vi "schedule.vi"(6 "Lighting Power Consume (W)":dbl format="%#_13g", 8 "Lenght of Light Period (hr)":i32, 9 "Start Time of Light Period":i32, 10 "input envTemp. & elecFee":cluster{"Temp.":dbl[], "elecFee":dbl[]}={"Temp."=[29.6, 26.5, 26.8, 26.8, 26.5, 26.9, 27.8, 28.5, 26.3, 30.1, 33.3, 33.4, 33.9, 32.2, 32.7, 32.7, 32.4, 31.5, 30.5, 29.7, 28.3, 28.2, 27.9, 27.5], "elecFee"=[2.2, 2.2, 2.2, 2.2, 2.2, 2.2, 2.2, 2.2, 3.5, 3.5, 3.5, 3.5, 3.5, 3.5, 3.5, 3.5, 3.5, 3.5, 3.5, 3.5, 3.5, 3.5, 2.2, 2.2]}, 11 "input Parameter":T2={"input COP of ACs"=3.0, "input setDay Temp"=22.0, "input setNight Temp."=20.0}) -> (3 "group Outcome":T1 {"group hourly total elecFee" format="%#.2g"; "group Total elecFee" format="%#.2g"; "group hourly ACs elecFee" format="%#.2g"; "group ACs elecFee" format="%#.2g"; "group hourly LEDs elecFee" format="%#.2g"; "group Total LEDs elecFee" format="%#.2g"})   [LabVIEW 2014]
panel:
  out "setNight Temp.":dbl
  out "setDay Temp.":dbl
  out "COP of ACs":dbl
  # "0~1"
  # "1~2"
  # "2~3"
  # "3~4"
  # "4~5"
  # "5~6"
  # "6~7"
  # "7~8"
  # "8~98~9"
  # "9~10"
  # "10~11"
  # "11~12"
  # "12~13"
  # "13~14"
  # "14~15"
  # "15~16"
  # "16~17"
  # "17~18"
  # "18~19"
  # "19~20"
  # "21~21"
  # "21~22"
  # "22~23"
  # "23~24"
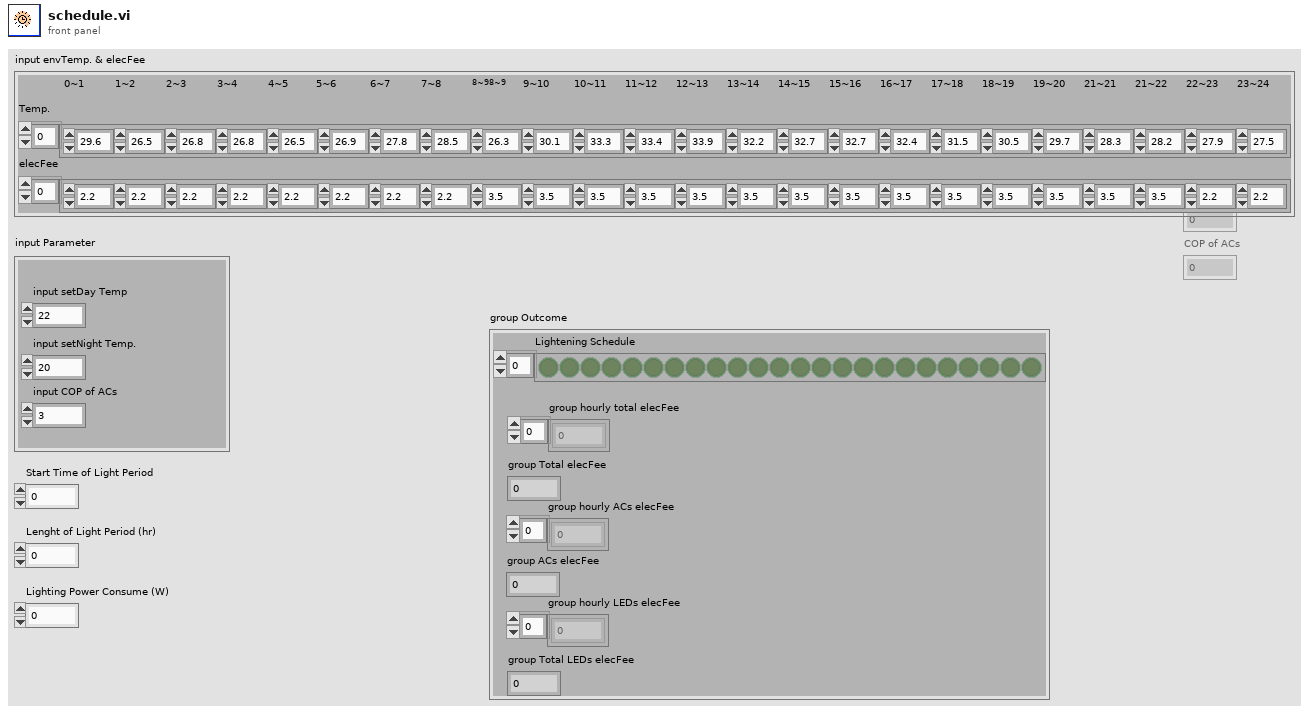
[diagram p1: front panel]
types:
  T1 = cluster{"Lightening Schedule":bool[], "group hourly total elecFee":dbl[], "group Total elecFee":dbl, "group hourly ACs elecFee":dbl[], "group ACs elecFee":dbl, "group hourly LEDs elecFee":dbl[], "group Total LEDs elecFee":dbl}
  T2 = cluster{"input COP of ACs":dbl, "input setDay Temp":dbl, "input setNight Temp.":dbl}
  T3 = cluster{bool[], dbl[], dbl, dbl[], dbl, dbl[], dbl}
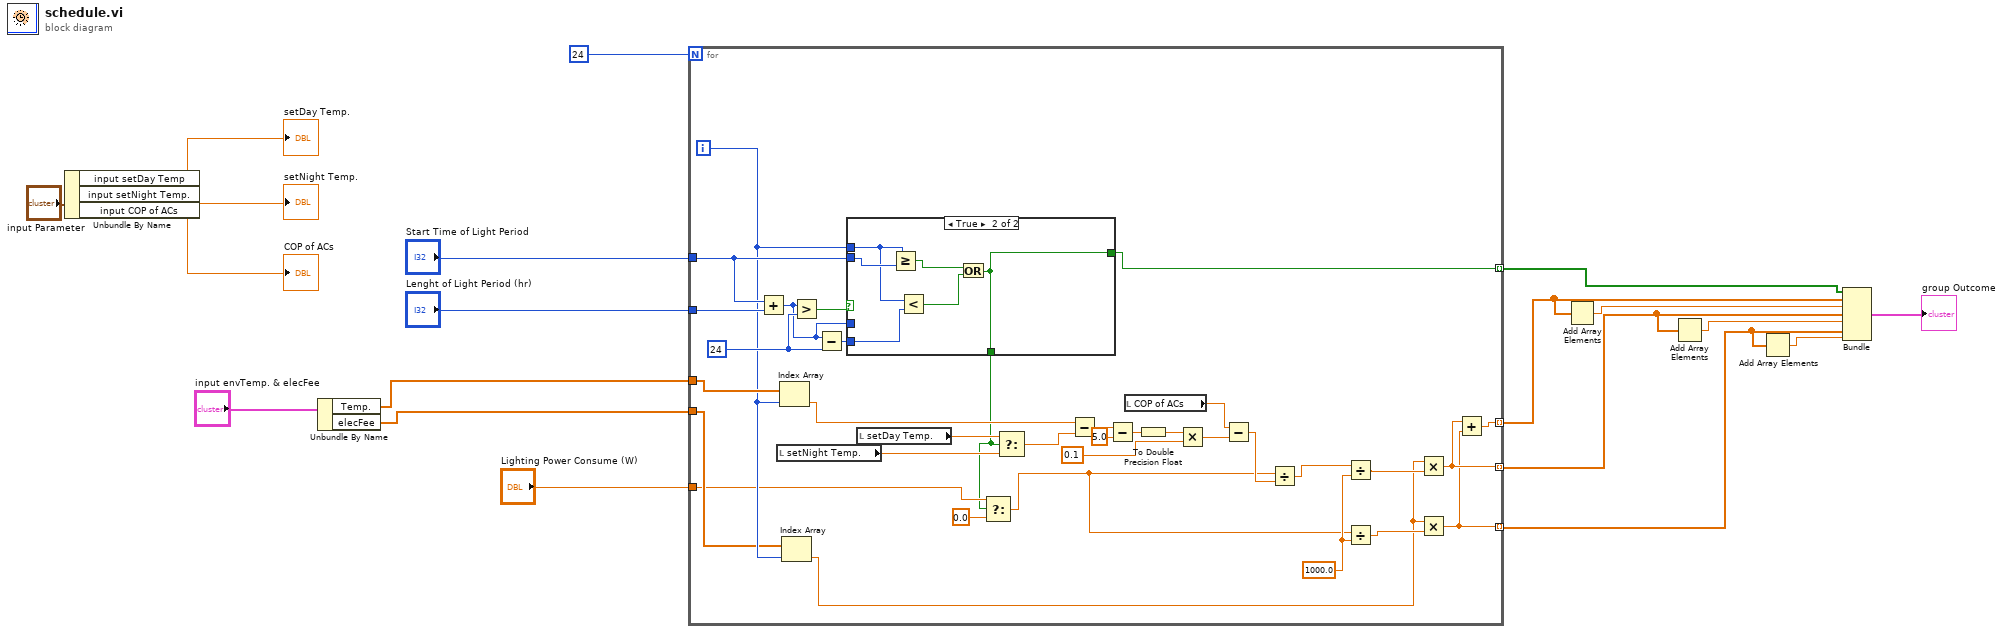
[diagram p0: block diagram]
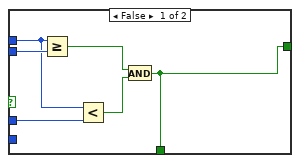
[diagram p2: hidden frame]
diagram:
  n1 = Unbundle By Name("input Parameter") -> ("input setDay Temp"=→"setDay Temp.":dbl, "input setNight Temp."=→"setNight Temp.":dbl, "input COP of ACs"=→"COP of ACs":dbl)
  n2 = Unbundle By Name("input envTemp. & elecFee") -> ("Temp."=w10:dbl[], "elecFee"=w9:dbl[])
  n3 = for {
    N: 24 ("Numeric") -> [_]
    tunnel: "Start Time of Light Period" -> [w51]
    tunnel: "Lenght of Light Period (hr)" -> [w53]
    tunnel: "Lighting Power Consume (W)" -> [w26]
    tunnel: [w23] -> w5 mode=indexing
    tunnel: [w22] -> w2 mode=indexing
    tunnel: w10 -> [w32]
    tunnel: w9 -> [w30]
    tunnel: [w20] -> w8 mode=indexing
    tunnel: [w21] -> w7 mode=indexing
    i -> [w31]
    w34 = 1000.0
    w50 = 24 ("y")
    n4 = Add(x=w51, y=w53) -> (x+y=w48:i32)
    n5 = local read "setNight Temp."() -> (w46:dbl)
    n6 = Index Array(array=w32, index=w31) -> (element=w29:dbl)
    n7 = Index Array(array=w30, index=w31) -> (element=w28:dbl)
    n8 = Greater?(x=w48, y=w50) -> (0:w52:bool)
    n9 = Subtract(x=w48, y=w50) -> (x-y=w49:i32)
    n10 = case shown="True" w52 {
      tunnel: w31 -> [w58 w61]
      tunnel: w51 -> [w59 w65]
      tunnel: [w54 w60] -> w20
      tunnel: w49 -> [_ w63]
      tunnel: w48 -> [w57 _]
      tunnel: [w54 w60] -> w25
      frame False {
        n11 = Greater Or Equal?(x=w58, y=w59) -> (x >= y?=w56:bool)
        n12 = Less?(x=w58, y=w57) -> (x < y?=w55:bool)
        n13 = And(x=w56, y=w55) -> (x .and. y?=w54:bool)
      }
      frame True {
        n14 = Greater Or Equal?(x=w61, y=w65) -> (x >= y?=w64:bool)
        n15 = Less?(x=w61, y=w63) -> (x < y?=w62:bool)
        n16 = Or(x=w64, y=w62) -> (x .or. y?=w60:bool)
      }
    }
    n17 = local read "setDay Temp."() -> (w47:dbl)
    n18 = Select(t=w26, s=w25, f=0.0) -> (s? t:f=w27:dbl)
    n19 = Select(t=w47, s=w25, f=w46) -> (s? t:f=w45:dbl)
    n20 = Subtract(x=w29, y=w45) -> (x-y=w44:dbl)
    n21 = Subtract(x=w44, y=5.0) -> (x-y=w39:dbl)
    n22 = local read "COP of ACs"() -> (w38:dbl)
    n23 = To Double Precision Float(number=w39) -> (double precision float=w40:dbl)
    n24 = Multiply(x=w40, y=0.1) -> (x*y=w41:dbl)
    n25 = Subtract(x=w38, y=w41) -> (x-y=w37:dbl)
    n26 = Divide(x=w27, y=w37) -> (x/y=w33:dbl)
    n27 = Divide(x=w33, y=w34) -> (x/y=w36:dbl)
    n28 = Divide(x=w27, y=w34) -> (x/y=w35:dbl)
    n29 = Multiply(x=w28, y=w36) -> (x*y=w23:dbl)
    n30 = Multiply(x=w28, y=w35) -> (x*y=w22:dbl)
    n31 = Add(x=w23, y=w22) -> (x+y=w21:dbl)
  }
  n32 = Add Array Elements(numeric array=w7) -> (sum=w6:dbl)
  n33 = Add Array Elements(numeric array=w5) -> (sum=w4:dbl)
  n34 = Add Array Elements(numeric array=w2) -> (sum=w3:dbl)
  n35 = Bundle(w8, w7, w6, w5, w4, w2, w3) -> (→"group Outcome":T3)  [unwired: 1 in]
